vi "Shutdown.vi"(8 "error in (no error)":errorcluster, 11 "DtoA in":refnum<class "Wavepond.lvclass">) -> (0 "error out":errorcluster, 3 "DtoA out":refnum<class "Wavepond.lvclass">)   [LabVIEW 2014, in "Wavepond.lvclass"]
uses:
  Wavepond.lvclass
  External Clock.lvclass
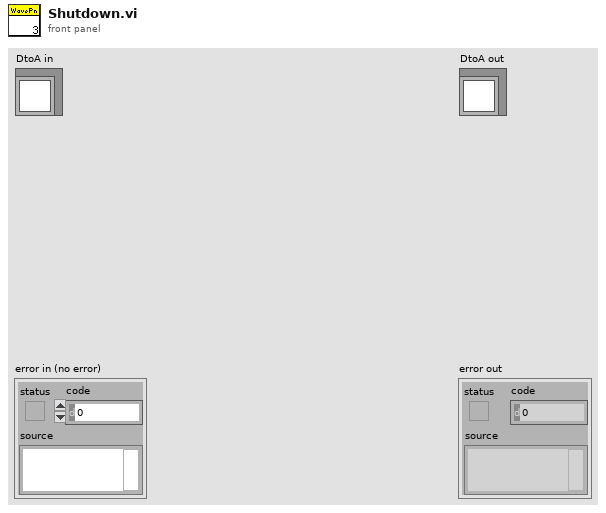
[diagram p1: front panel]
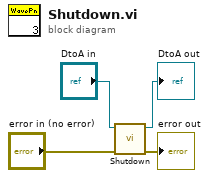
[diagram p0: block diagram]
diagram:
  n1 = call-parent "Shutdown.vi"("error in (no error)"="error in (no error)", "DtoA in"="DtoA in") -> ("error out"=→"error out":errorcluster, "DtoA out"=→"DtoA out":refnum<class "Wavepond.lvclass">)  [unwired: 8 in]
